vi "adlink7230Close.vi"(8 "error in (no error)":errorcluster caption="错误输入（无错误）", 10 "task in Output":refnum<k7>, 11 "task in Input":refnum<k7>) -> (0 "error out":errorcluster caption="错误输出")   [LabVIEW 2017]
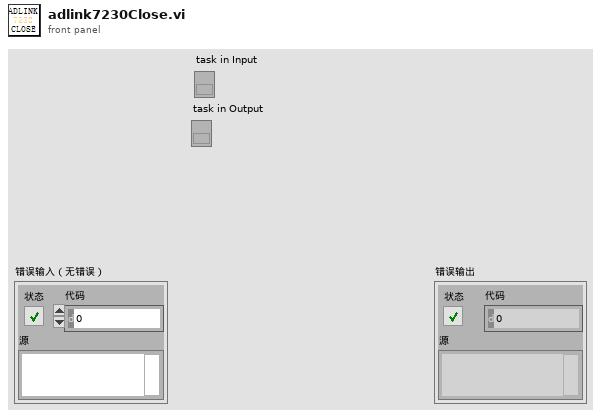
[diagram p1: front panel]
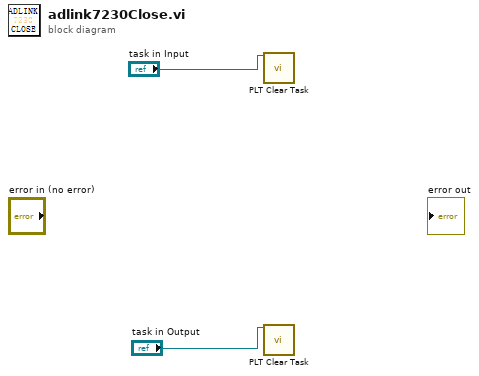
[diagram p0: block diagram]
diagram:
  n1 = call <userlib>:"PLT Clear Task.vi"("task in"="task in Input") -> ()  [unwired: 14 in, 1 out]
  n2 = call <userlib>:"PLT Clear Task.vi"("task in"="task in Output") -> ()  [unwired: 14 in, 1 out]
